vi "MotorControl_4channelDigitalOut.vi"(0 "Channel 1":tag, 1 "Channel 2":tag, 2 "Motor Position Control":dbl, 3 "Channel 3":tag, 4 "Channel 4":tag) -> (5 "error out":errorcluster)   [LabVIEW 2015]
doc: "Motor control--4 digital output channel\n=====================\n\nInput\n------\nMotor Position Control: Position of Motor to be turned\nChannel 1, Channel 2, Channel 3 and Channel 4: Digital output pin\n\nOutput\n--------\nerror out: Error"
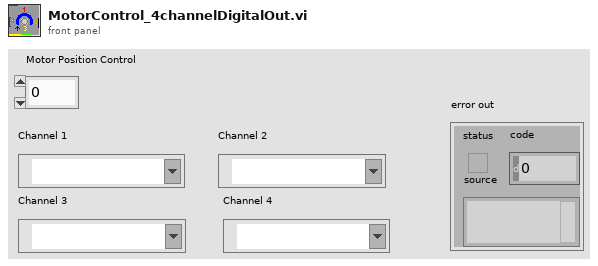
[diagram p1: front panel]
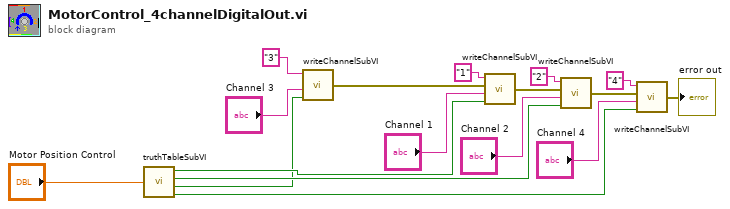
[diagram p0: block diagram]
diagram:
  n1 = call "truthTableSubVI.vi"("Numeric"="Motor Position Control") -> ("Boolean"=w7:bool, "Boolean 2"=w6:bool, "Boolean 3"=w5:bool, "Boolean 4"=w4:bool)
  n2 = call "writeChannelSubVI.vi"("data"=w5, "lines"="Channel 3", "name to assign"="3" ("name to assign 4")) -> ("error out"=w3:errorcluster)  [unwired: 1 in]
  n3 = call "writeChannelSubVI.vi"("data"=w7, "lines"="Channel 1", "error in"=w3, "name to assign"="1") -> ("error out"=w2:errorcluster)
  n4 = call "writeChannelSubVI.vi"("data"=w6, "lines"="Channel 2", "error in"=w2, "name to assign"="2" ("name to assign 3")) -> ("error out"=w1:errorcluster)
  n5 = call "writeChannelSubVI.vi"("data"=w4, "lines"="Channel 4", "error in"=w1, "name to assign"="4" ("name to assign 2")) -> ("error out"=→"error out":errorcluster)
